vi "Turn-Degrees-Subtask1.vi"() -> ()   [LabVIEW 2016, in "LEGO-PMR.lvrbt"]
uses:
  LEGO-PMR.lvrbt
  <vilib>/NXT/Block Support/NXT_InputPort.ctl
  <vilib>/NXT/Block Support/NXT_OutputPort.ctl
  <vilib>/NXT/Dual Mode Library/Sensors/EV3_Ultrasonic_CM.vi
  <vilib>/NXT/NXTIO Xnodes/NXTIONodeSubVIs/NXTMoveMotors.vi
  <vilib>/NXT/Dual Mode Library/Waits/Wait_Num.vi
  <vilib>/NXT/NXTIO Xnodes/AddressXNode/NXTIOAddress.xnode
  <vilib>/NXT/NXTIO Xnodes/NXTIOXNode/NXTIO.xnode
  <vilib>/NXT/Subs/LVHSConnector.ctl
  <vilib>/NXT/LegoClasses/BrickReference/BrickReference.lvclass
panel:
  in  "Distance to object marker":dbl
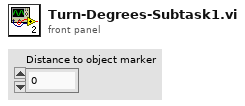
[diagram p1: front panel]
types:
  T1 = typedef "NXT_OutputPort.ctl" = u8
  T2 = typedef "NXT_InputPort.ctl" = u32
  T3 = typedef "LVHSConnector.ctl" = refnum<class "BrickReference.lvclass">
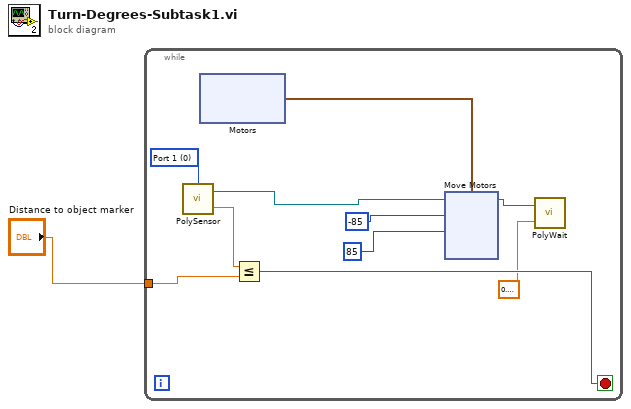
[diagram p0: block diagram]
diagram:
  n1 = while {
    tunnel: "Distance to object marker" -> [w10]
    stop <- w8 stop-if-true
    w2 = T2 0 items=["Port 1", "Port 2", "Port 3", "Port 4"] ("Port (Port 1)")
    n2 = call-poly <vilib>:"PolySensor.vi"("Port (Port 1)"=w2) -> ("Centimeters"=w9:sgl, "NXT/EV3"=w7:T3)  [unwired: 2 in]
    n3 = xnode "Motors"() -> ("Motor"=w11:cluster{"Port":T1, "Port":T1})
    n4 = Less Or Equal?(x=w9, y=w10) -> (x <= y?=w8:bool)
    n5 = xnode "Move Motors"("Power/Speed 2"=85, "Power/Speed 1"=-85, "Motors"=w11, "NXT/EV3"=w7) -> ("NXT/EV3"=w4:T3)
    n6 = call-poly <vilib>:"PolyWait.vi"("Time (1 sec)"=0.10000000000000002, "NXT/EV3"=w4) -> ()  [unwired: 2 in, 1 out]
  }
